vi "ScvmmTriggerClientHemanth.vi"() -> ()   [LabVIEW 2020]
panel:
  out "stop":bool
  out "CMD output":string
  out "Consumer error":errorcluster
  out "Message Log:":string
  out "Ghost Server Name":string="devimageserver"
  out "Producer error":errorcluster
  out "Ghost Server IP":string
  out "Listening on Port:":u16=5555
  # "DO NOT STOP OR CLOSE THIS APP!"
  # "This utility allows remote triggering of existing Ghost tasks and is used by external schedulers.\nTo use this to remotely trigger your tasks, add the following to your external application:\n\n1) Open a TCP connection with the Ghost Server IP or name and Port listed below.\n2) Send a string containing nothing but the VM name you want to execute:\n     (e.g. \"rtvm01a\").  For backwards compatibility, \"rtvm01a\\ATS Test\" will be read as \"rtvm01a.\"\nThis program runs the PowerShell script here: C:\\RevertCheckpoint.ps1"
  # "This utility is owned by Brian Frantz (LabVIEW RT)."
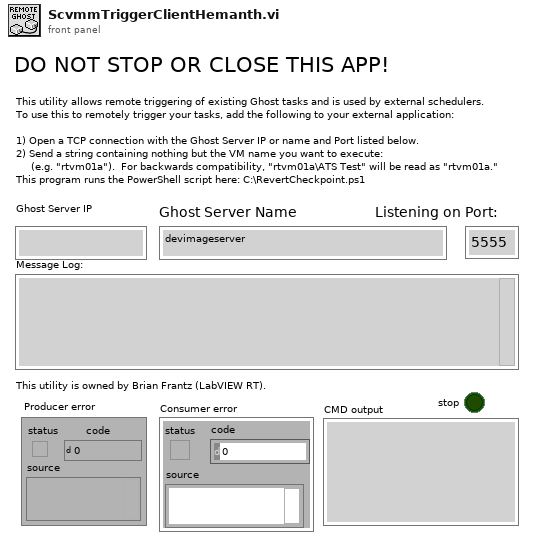
[diagram p1: front panel]
types:
  T1 = enum16{"Standard", "Buffered", "CRLF", "Immediate"}
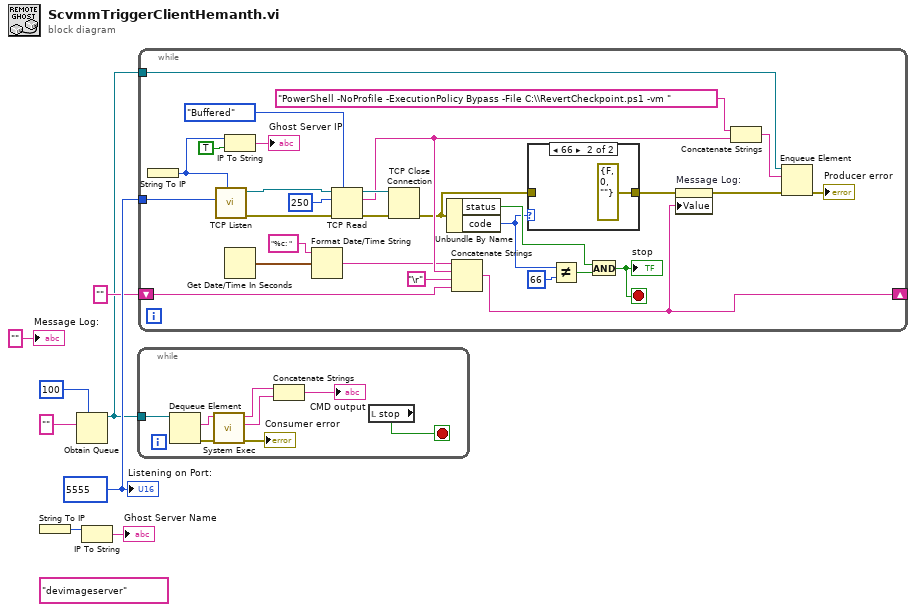
[diagram p0: block diagram]
diagram:
  w8 = u16 5555 ("port")
  (unwired) "devimageserver"
  n1 = String To IP() -> (0:w5:u32)  [unwired: 1 in]
  n2 = Obtain Queue(max queue size (-1, unlimited)=100, element data type="" ("name")) -> (queue out=w2:refnum<queue>)  [unwired: 3 in, 2 out]
  n3 = IP To String(2:w5) -> (0:→"Ghost Server Name":string)  [unwired: 1 in]
  n4 = while {
    tunnel: w2 -> [w16]
    stop <- w9 stop-if-true
    n5 = Dequeue Element(queue=w16) -> (element=w13:string, error out=w15:errorcluster)  [unwired: 2 in, 2 out]
    n6 = call <vilib>:"System Exec.vi"("error in (no error)"=w15, "command line"=w13) -> ("error out"=→"Consumer error":errorcluster, "standard error"=w11:string, "standard output"=w12:string)  [unwired: 6 in, 1 out]
    n7 = Concatenate Strings(w12, w11) -> (→"CMD output":string)
    n8 = local read "stop"() -> (w9:bool)
  }
  n9 = while {
    tunnel: w8 -> [w31]
    shift-right: [w22] -> _
    shift-left: "" ("string") -> [w24]
    tunnel: w2 -> [w19]
    stop <- w33 stop-if-true
    n10 = String To IP() -> (0:w39:u32)  [unwired: 1 in]
    n11 = call <vilib>:"TCP Listen.vi"("net address"=w39, "port"=w31) -> ("error out"=w42:errorcluster, "connection ID"=w41:refnum<k5>)  [unwired: 5 in, 3 out]
    n12 = IP To String(1:TRUE ("dot notation? (F)"), 2:w39) -> (0:→"Ghost Server IP":string)
    n13 = Get Date/Time In Seconds() -> (seconds since 1Jan1904=w23:timestamp)
    n14 = Format Date/Time String(time format string (%c)="%c: ", seconds (now)=w23) -> (date/time string=w28:string)  [unwired: 1 in]
    n15 = TCP Read(connection ID=w41, bytes to read=250, error in (no error)=w42, 7:T1."Buffered" ("mode (standard)")) -> (connection ID out=w45:refnum<k5>, data out=w29:string, error out=w44:errorcluster)  [unwired: 1 out]
    n16 = TCP Close Connection(connection ID=w45, error in (no error)=w44) -> (error out=w25:errorcluster)  [unwired: 2 out]
    n17 = Unbundle By Name(w25) -> ("status"=w35:bool, "code"=w30:i32)
    n18 = Concatenate Strings(w28, w29, "\r", w24) -> (w22:string)
    n19 = case shown="66" w30 {
      tunnel: w25 -> [w46 _]
      tunnel: [w46 errorcluster {"status"=FALSE, "code"=0, "source"=""} ("error out")] -> w21
      frame 0, Default {
      }
      frame 66 {
      }
    }
    n20 = Not Equal?(x=w30, y=66) -> (x != y?=w34:bool)
    n21 = And(x=w35, y=w34) -> (x .and. y?=w33:bool)
    "stop" <- w33
    n22 = property on="Message Log:" class="Str"(error in=w21, "Value"=w22) -> (error out=w18:errorcluster)  [unwired: 1 in, 1 out]
    n23 = Concatenate Strings("PowerShell -NoProfile -ExecutionPolicy Bypass -File C:\\RevertCheckpoint.ps1 -vm " ("string"), w29) -> (w20:string)
    n24 = Enqueue Element(queue=w19, element=w20, error in (no error)=w18) -> (error out=→"Producer error":errorcluster)  [unwired: 1 in, 2 out]
  }
  "Listening on Port:" <- w8
  "Message Log:" <- "" ("Message Log:")
